vi "Get EtherCAT Slave refs.vi"(8 "error in (no error)":errorcluster, 11 "Ip address":string) -> (0 "error out":errorcluster, 3 "Slave Refs":refnum<k21>[](array[refnum]))   [LabVIEW 2016, in "ds402mgr_Helper.lvlib"]
uses:
  ds402mgr_Helper.lvlib
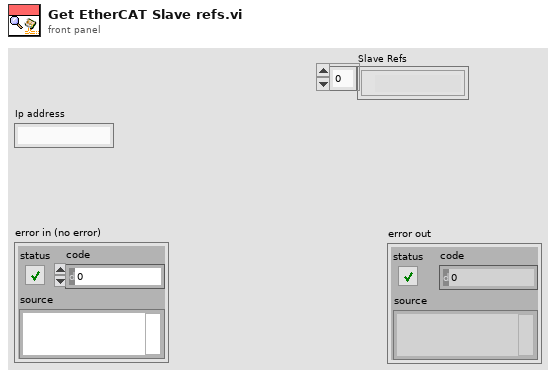
[diagram p1: front panel]
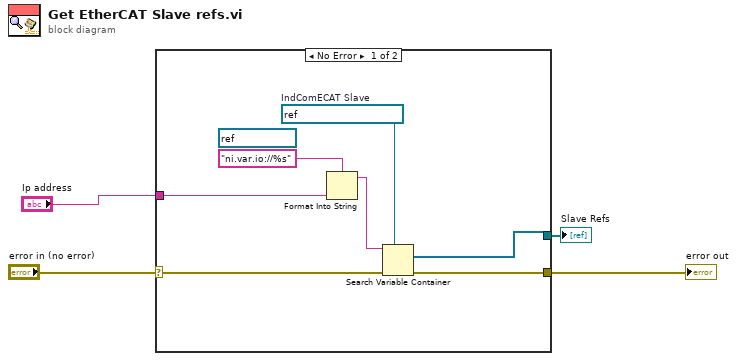
[diagram p0: block diagram]
diagram:
  n1 = case shown="No Error" "error in (no error)" {
    selector: "error in (no error)" -> [w8 w12]
    tunnel: "Ip address" -> [w6 _]
    tunnel: [w7 w12] -> w2
    tunnel: [w5 _] -> w1
    frame No Error {
      (unwired) refnum<k21> "ni.var.io:/" ("container refnum in")
      w9 = refnum<k21> refnum  # IndComECAT Slave
      n2 = Format Into String(format string="ni.var.io://%s", w6) -> (resulting string=w11:string)  [unwired: 2 in, 1 out]
      n3 = Search Variable Container(7:w9, 8:w8, 11:w11) -> (0:w7:errorcluster, 2:w5:refnum<k21>[])  [unwired: 3 in, 1 out]
    }
    frame Error {
    }
  }
  "error out" <- w2
  "Slave Refs" <- w1
